vi "Demo.vi"() -> ()   [LabVIEW 2018]
doc: "This will prevent the system from sleeping when run and will prevent the screen-saver from turning on when the mouse is hovered over the 'Keep Screen On' button."
uses:
  Power Availabilty Requests/Type Defs/Power Request Type.ctl
  <vilib>/Utility/inputDevices.llb/closeMouse.vi
  Power Requests.lvlib
panel:
  in  "stop":bool
  in  "Keep Screen On":bool
  # "Overview: This will prevent the system from sleeping when run and will prevent the screen-saver from turning on when the mouse is hovered over the Keep Screen On button.\nRequirements: LabVIEW 2012 (or compatible)\nInstructions: \n1. Run this VI"
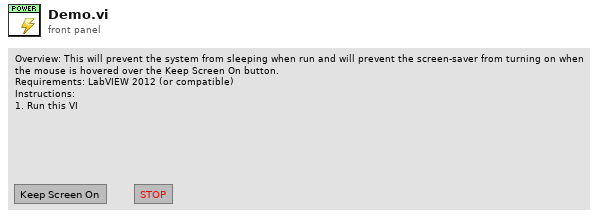
[diagram p1: front panel]
types:
  T1 = typedef "Power Requests.lvlib/Power Request Type.ctl" = enum32{"Power Request Display Required", "Power Request System Required", "Power Request Away Mode Required", "Power Request Execution Required"}
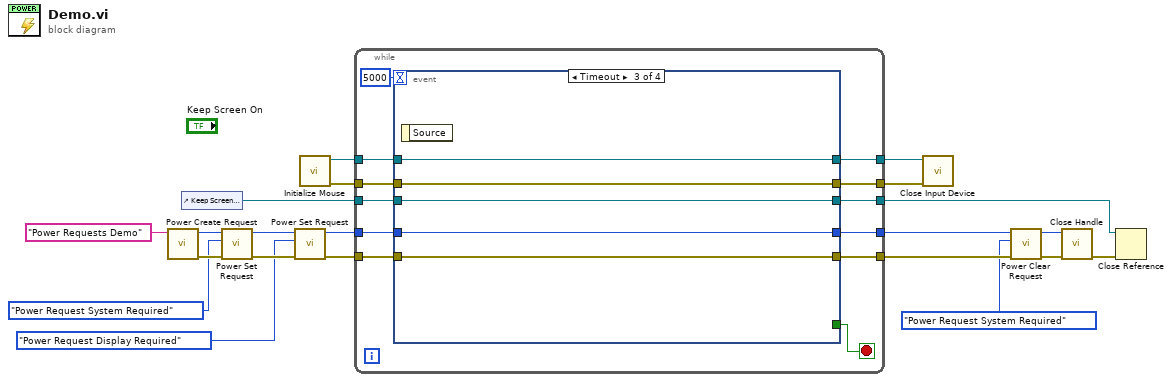
[diagram p0: block diagram]
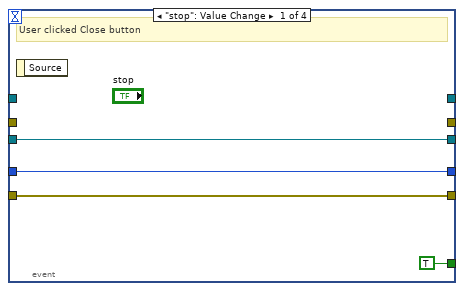
[diagram p2: hidden frame]
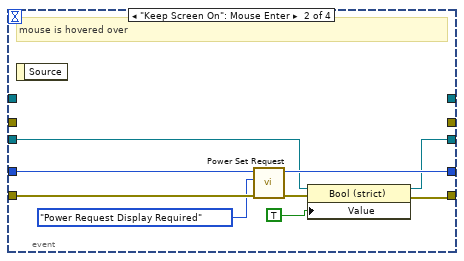
[diagram p3: hidden frame]
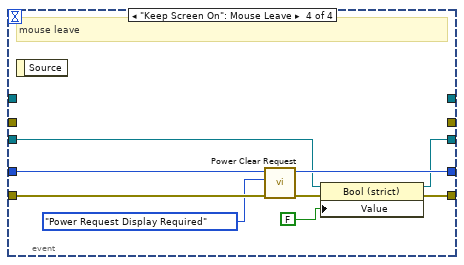
[diagram p4: hidden frame]
diagram:
  n1 = call "Power Create Request.vi"("Simple Reason String"="Power Requests Demo") -> ("error out"=w21:errorcluster, "Handle"=w20:i64)  [unwired: 9 in]
  n2 = control-ref of="Keep Screen On"() -> (w11:refnum<vi>)
  n3 = call "Power Set Request.vi"("error in (no error)"=w21, "Power Request Type"=Power_Request_Type."Power Request System Required", "Handle in"=w20) -> ("error out"=w19:errorcluster, "Handle out"=w7:u32)  [unwired: 6 in, 1 out]
  n4 = call "Power Set Request.vi"("error in (no error)"=w19, "Power Request Type"=Power_Request_Type."Power Request Display Required", "Handle in"=w7) -> ("error out"=w8:errorcluster, "Handle out"=w6:u32)  [unwired: 6 in, 1 out]
  n5 = call <vilib>:"Initialize Mouse.vi"() -> ("error out"=w3:errorcluster, "device ID"=w4:refnum<k1>)  [unwired: 10 in]
  n6 = while {
    tunnel: w8 -> [w32]
    tunnel: [w31] -> w18
    tunnel: w6 -> [w30]
    tunnel: [w29] -> w12
    tunnel: w11 -> [w28]
    tunnel: [w27] -> w9
    tunnel: w4 -> [w26]
    tunnel: w3 -> [w25]
    tunnel: [w23] -> w2
    tunnel: [w22] -> w1
    stop <- w33 stop-if-true
    n7 = event shown="[2] Timeout" {
      selector: _ -> [_ _ _ _]
      dyn-events: _ -> [_ _ _ _]
      timeout: 5000 -> [_ _ _ _]
      tunnel: [TRUE _ _ _] -> w33
      tunnel: w32 -> [w37 w44 w49 w60]
      tunnel: [w37 w41 w49 w55] -> w31
      tunnel: w30 -> [w36 w46 w50 w59]
      tunnel: [w36 w45 w50 w58] -> w29
      tunnel: w28 -> [w35 w40 w51 w54]
      tunnel: [w35 w39 w51 w53] -> w27
      tunnel: w26 -> [_ _ w48 _]
      tunnel: w25 -> [_ _ w47 _]
      tunnel: [_ _ w48 _] -> w23
      tunnel: [_ _ w47 _] -> w22
      event "stop": Value Change {
        # "User clicked Close button"
        n8 = event-data() -> ()  [unwired: 1 in, 1 out]
      }
      event "Keep Screen On": Mouse Enter {
        # "mouse is hovered over"
        n9 = event-data() -> ()  [unwired: 1 in, 1 out]
        n10 = call "Power Set Request.vi"("error in (no error)"=w44, "Power Request Type"=Power_Request_Type."Power Request Display Required", "Handle in"=w46) -> ("error out"=w42:errorcluster, "Handle out"=w45:u32)  [unwired: 6 in, 1 out]
        n11 = property class="Bool (strict)"(reference=w40, error in=w42, "Value"=TRUE) -> (reference out=w39:refnum<vi>, error out=w41:errorcluster)
      }
      event Timeout {
        n12 = event-data() -> ()  [unwired: 1 in, 1 out]
      }
      event "Keep Screen On": Mouse Leave {
        # "mouse leave"
        n13 = event-data() -> ()  [unwired: 1 in, 1 out]
        n14 = call "Power Clear Request.vi"("error in (no error)"=w60, "Power Request Type"=Power_Request_Type."Power Request Display Required", "Handle in"=w59) -> ("error out"=w56:errorcluster, "Handle out"=w58:u32)  [unwired: 6 in, 1 out]
        n15 = property class="Bool (strict)"(reference=w54, error in=w56, "Value"=FALSE) -> (reference out=w53:refnum<vi>, error out=w55:errorcluster)
      }
    }
  }
  n16 = call-poly <vilib>:"Close Input Device.vi"("error in (no error)"=w1, "device ID"=w2) -> ()  [unwired: 8 in, 1 out]
  n17 = call "Power Clear Request.vi"("error in (no error)"=w18, "Power Request Type"=Power_Request_Type."Power Request System Required", "Handle in"=w12) -> ("error out"=w17:errorcluster, "Handle out"=w16:u32)  [unwired: 6 in, 1 out]
  n18 = call "Close Handle.vi"("error in (no error)"=w17, "Handle"=w16) -> ("error out"=w10:errorcluster)  [unwired: 8 in, 1 out]
  n19 = Close Reference(reference=w9, error in (no error)=w10) -> ()  [unwired: 1 out]
